vi "Quench.vi"(8 "Error In":errorcluster, 10 "Quench":bool, 11 "KIT-QVA in":refnum<class "KIT-QVA.lvclass">) -> (0 "Error Out":errorcluster, 3 "KIT-QVA out":refnum<class "KIT-QVA.lvclass">)   [LabVIEW 2014, in "KIT-QVA.lvlib" / "KIT-QVA.lvclass"]
doc: "Stop control mode of QVision, equivalent to a quench event."
uses:
  KIT-QVA.lvclass
  KIT-QVA.lvclass/KIT-QVA.ctl
  CSPP_Core/Actors/CS++BaseActor/CS++BaseActor.lvclass/CS++BaseActor.ctl
  instr.lib/KIT-QV/KIT QV.lvlib
  CSPP_Core/Libraries/Utilities/CS++Utilities.lvlib
  CSPP_Core/Actors/CS++BaseActor/CS++BaseActor.lvclass
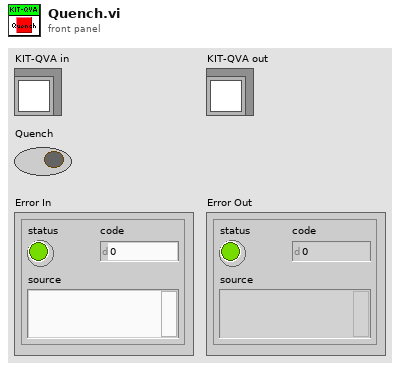
[diagram p1: front panel]
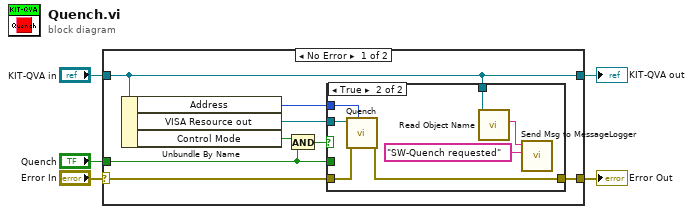
[diagram p0: block diagram]
diagram:
  n1 = case shown="No Error" "Error In" {
    selector: "Error In" -> [w11 w23]
    tunnel: [w10 w23] -> w4
    tunnel: [w6 w22] -> w2
    tunnel: "KIT-QVA in" -> [w6 w22]
    tunnel: "Quench" -> [w7 _]
    frame No Error {
      n2 = Unbundle By Name(w6) -> ("Address"=w12:u16, "VISA Resource out"=w13:refnum<visa-resource-name>, "Control Mode"=w9:bool)
      n3 = And(x=w9, y=w7) -> (x .and. y?=w8:bool)
      n4 = case shown="True" w8 {
        tunnel: w13 -> [_ w21]
        tunnel: w12 -> [_ w20]
        tunnel: w11 -> [w14 w19]
        tunnel: w7 -> [_ _]
        tunnel: [w14 w18] -> w10
        tunnel: w6 -> [_ w15]
        frame False {
        }
        frame True {
          n5 = call "Quench.vi"("Address"=w20, "Error In"=w19, "VISA Resource in"=w21) -> ("Error Out"=w18:errorcluster)  [unwired: 7 in, 1 out]
          n6 = call "Read Object Name.vi"("CS++BaseActor in"=w15) -> ("Object Name"=w16:string)  [unwired: 8 in, 2 out]
          n7 = call "Send Msg to MessageLogger.vi"("Message Content"="SW-Quench requested", "Message Tag"=w16) -> ()  [unwired: 9 in, 1 out]
        }
      }
    }
    frame Error {
    }
  }
  "Error Out" <- w4
  "KIT-QVA out" <- w2
